vi "TPG366_get_p_all.vi"(8 "error in":errorcluster, 11 "conn_in":refnum<k5>) -> (0 "err_out":errorcluster, 1 "pressure":dbl[](array[numeric]) caption="Torr" format="%_5e", 2 "status":i8[](array[numeric]), 3 "conn_out":refnum<k5>, 4 "status_comm":bool)   [LabVIEW 2019]
panel:
  in  "timeout":i32=100
  out "bytes written":i32
  out "read_2":string
  out "read_1":string
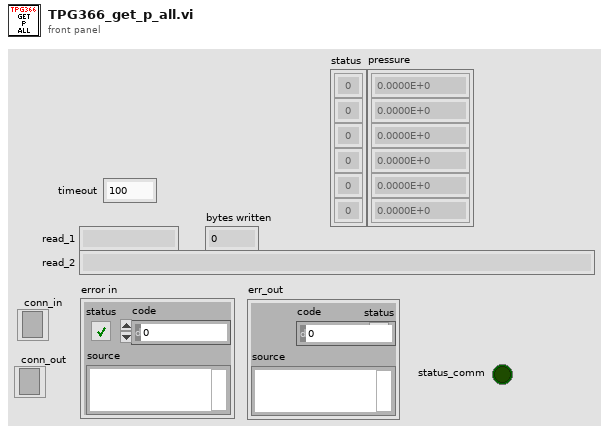
[diagram p1: front panel]
types:
  T1 = enum16{"Standard", "Buffered", "CRLF", "Immediate"}
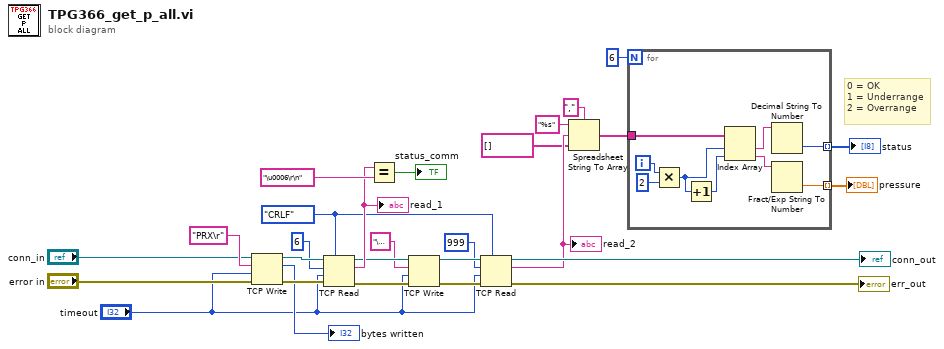
[diagram p0: block diagram]
diagram:
  w9 = T1."CRLF" ("mode (standard)")
  # "0 = OK\n1 = Underrange\n2 = Overrange"
  n1 = TCP Write(connection ID="conn_in", data in="PRX\r" ("string"), error in (no error)="error in", 9:"timeout") -> (connection ID out=w25:refnum<k5>, bytes written=→"bytes written":i32, error out=w24:errorcluster)
  n2 = TCP Read(connection ID=w25, bytes to read=6, error in (no error)=w24, 7:w9, 9:"timeout") -> (connection ID out=w19:refnum<k5>, data out=w20:string, error out=w18:errorcluster)
  "read_1" <- w20
  n3 = Equal?(x=w20, y="\u0006\r\n") -> (x = y?=→"status_comm":bool)
  n4 = TCP Write(connection ID=w19, data in="\u0005", error in (no error)=w18, 9:"timeout") -> (connection ID out=w16:refnum<k5>, error out=w15:errorcluster)  [unwired: 1 out]
  n5 = TCP Read(connection ID=w16, bytes to read=999, error in (no error)=w15, 7:w9, 9:"timeout") -> (connection ID out=→"conn_out":refnum<k5>, data out=w8:string, error out=→"err_out":errorcluster)
  "read_2" <- w8
  n6 = Spreadsheet String To Array(delimiter (Tab)="," ("search string/char (-)"), format string="%s", spreadsheet string=w8, array type (2D Dbl)=string[] [] ("format string")) -> (array=w4:string[])
  n7 = for {
    N: 6 -> [_]
    tunnel: w4 -> [w35]
    tunnel: [w30] -> w1 mode=indexing
    tunnel: [w29] -> w2 mode=indexing
    i -> [w37]
    n8 = Multiply(x=w37, y=2) -> (x*y=w34:i32)
    n9 = Increment(x=w34) -> (x+1=w33:i32)
    n10 = Index Array(array=w35, index #1=w34, index #2=w33) -> (element #1=w32:string, element #2=w31:string)
    n11 = Decimal String To Number(string=w32) -> (number=w30:i32)  [unwired: 2 in, 1 out]
    n12 = Fract/Exp String To Number(string=w31) -> (number=w29:dbl)  [unwired: 3 in, 1 out]
  }
  "pressure" <- w2
  "status" <- w1
